vi "CLL (SubVI).vi"(1 "Time cell\nnot used(months)":dbl, 2 "temperature IN":dbl) -> (0 "calendar life losses(%)":dbl)   [LabVIEW 2017]
panel:
  # "CLL = % CALENDAR LIFE LOSSES"
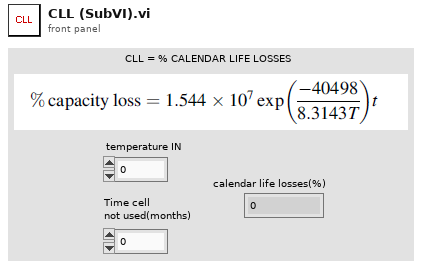
[diagram p1: front panel]
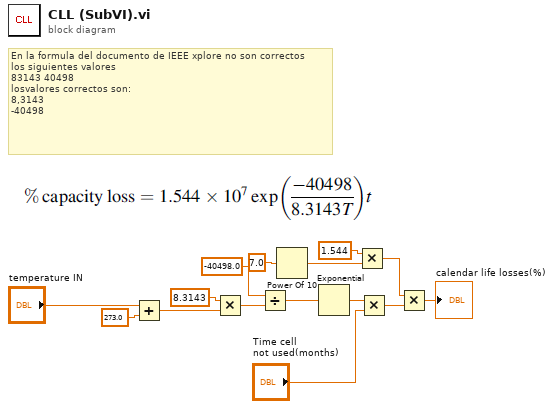
[diagram p0: block diagram]
diagram:
  # "En la formula del documento de IEEE xplore no son correctos\nlos siguientes valores \n83143 40498\nlosvalores correctos son:\n8,3143\n-40498"
  n1 = Add(x="temperature IN", y=273.0) -> (x+y=w3:dbl)
  n2 = Multiply(x=8.3143, y=w3) -> (x*y=w9:dbl)
  n3 = Divide(x=-40498.0, y=w9) -> (x/y=w7:dbl)
  n4 = Power Of 10(x=7.0) -> (10^x=w14:dbl)
  n5 = Exponential(1:w7) -> (0:w6:dbl)
  n6 = Multiply(x=1.544, y=w14) -> (x*y=w13:dbl)
  n7 = Multiply(x=w6, y="Time cell\nnot used(months)") -> (x*y=w4:dbl)
  n8 = Multiply(x=w13, y=w4) -> (x*y=→"calendar life losses(%)":dbl)
